vi "ReplaceVariantArrayElementBy1DIndex.vi"(9 "Index (1D)":u32, 10 "Value":variant, 11 "Array in":variant) -> (3 "Array out":variant)   [LabVIEW 2017]
uses:
  <vilib>/Utility/Data Type/NI_Data Type.lvlib
panel:
  out "Name":string
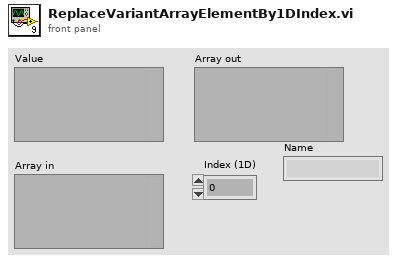
[diagram p1: front panel]
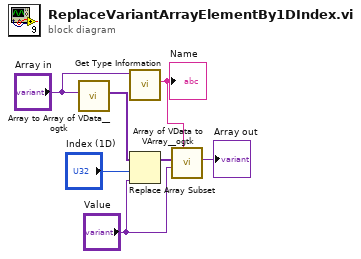
[diagram p0: block diagram]
diagram:
  n1 = call <userlib>:"Array to Array of VData__ogtk.vi"("MultiD Array"="Array in") -> ("1D Array of Variants"=w7:variant[])  [unwired: 9 in, 1 out]
  n2 = call <vilib>:"Get Type Information.vi"("Variant"="Array in") -> ("Name"=w2:string)  [unwired: 6 in, 4 out]
  "Name" <- w2
  n3 = Replace Array Subset(array=w7, new element="Value", index="Index (1D)") -> (w5:variant[])
  n4 = call <userlib>:"Array of VData to VArray__ogtk.vi"("Array Name"=w2, "Element Type (when empty)"="Value", "1D Array of VData"=w5) -> ("VArray"=→"Array out":variant)  [unwired: 7 in, 1 out]
